vi "SALVA COLLAUDO.vi"(5 "SALVA SOLO BOLLETTINO":bool, 6 "set valvole utilizzato":string[](array[string])=["-", "-", "-"], 7 "banco":string, 8 "Filtro":bool[](array[boolean]), 9 "SPECIALI?":bool[](array[boolean]), 10 "appended array":refnum<vi>[](array[refnum]), 11 "bollettino":string[][](array[string])) -> (2 "Collaudi ultimo salvataggio":string[](array[string]), 3 "NUMERO":string)   [LabVIEW 2019]
uses:
  <vilib>/addons/database/Connection.llb/Conn Execute.vi
  <vilib>/addons/database/Recordset.llb/Rec Fetch Recordset Data (R).vi
  <vilib>/addons/database/Recordset.llb/Rec Destroy - Connection.vi
  Global ricalcola progressivo salvataggio.vi
  <vilib>/addons/database/NI_Database_API.lvlib
panel:
  out "columns":string[](array[string])
  out "appended array 2":string[](array[string])
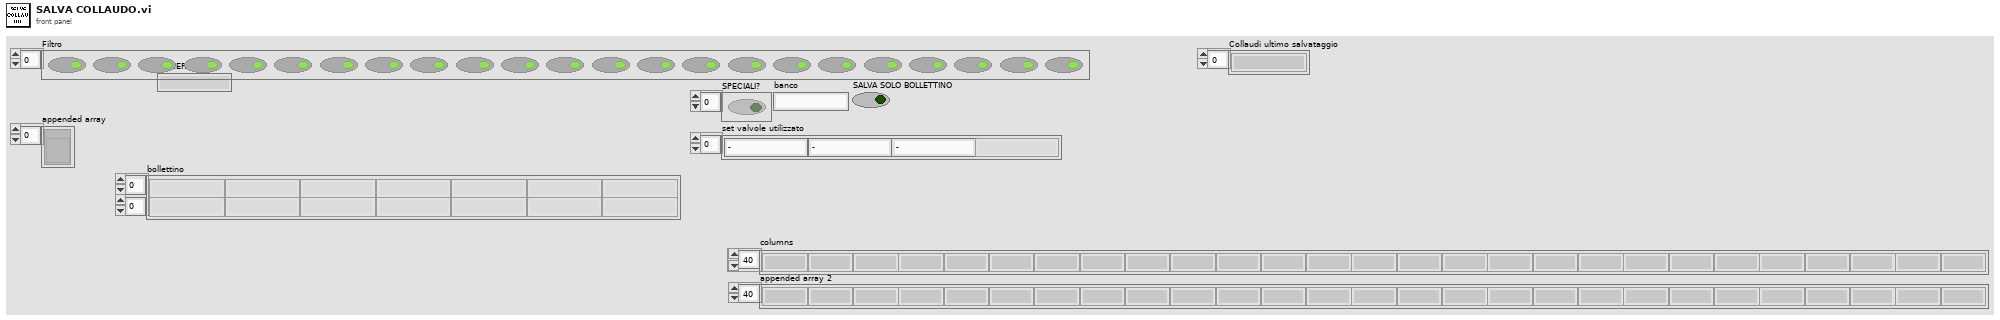
[diagram p1: front panel]
types:
  T1 = typedef "NI_Database_API.lvlib/Conn ObjectReference.ctl" = refnum<k1>
  T2 = typedef "NI_Database_API.lvlib/Rec ObjectReference.ctl" = refnum<k1>
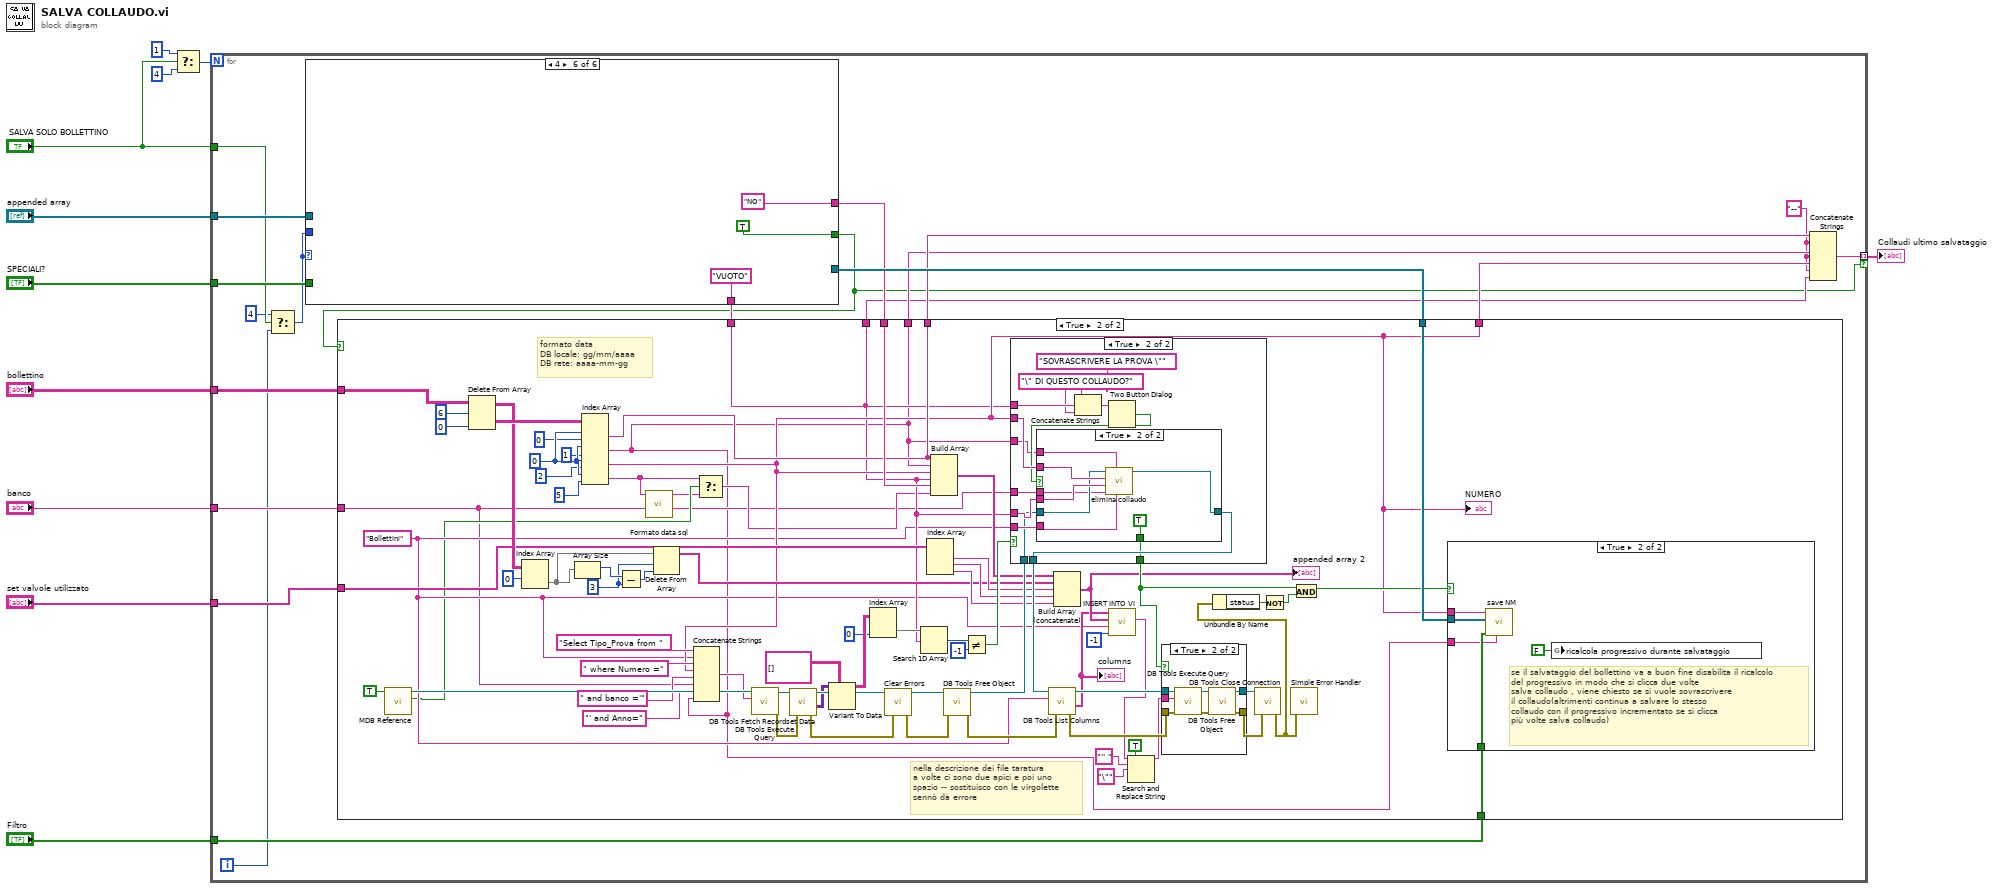
[diagram p0: block diagram]
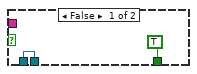
[diagram p5: hidden frame]
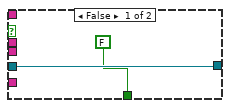
[diagram p6: hidden frame]
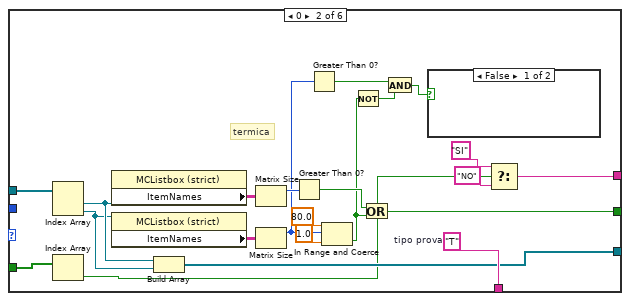
[diagram p8: hidden frame]
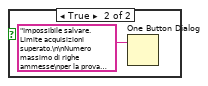
[diagram p9: hidden frame]
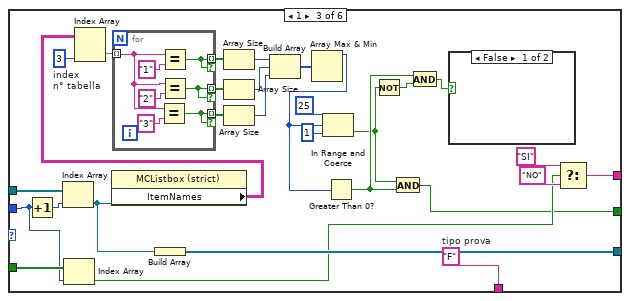
[diagram p10: hidden frame]
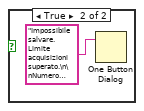
[diagram p11: hidden frame]
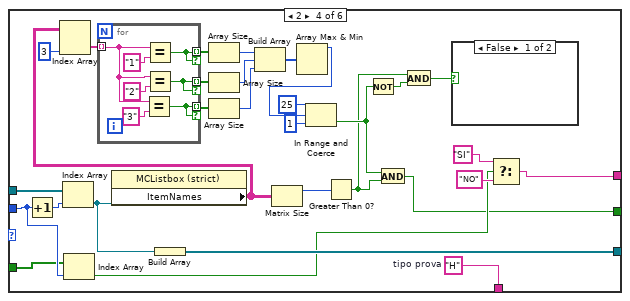
[diagram p12: hidden frame]
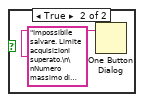
[diagram p13: hidden frame]
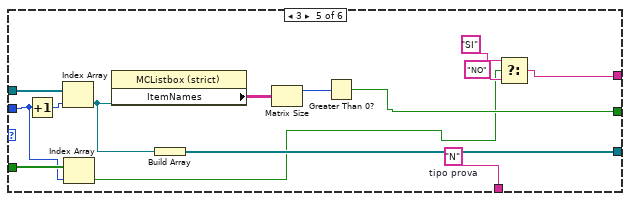
[diagram p14: hidden frame]
diagram:
  n1 = Select(t=1, s="SALVA SOLO BOLLETTINO", f=4) -> (s? t:f=w3:i32)
  n2 = for {
    N: w3 -> [_]
    tunnel: "bollettino" -> [w31]
    tunnel: "appended array" -> [w30]
    tunnel: "Filtro" -> [w27]
    tunnel: "SPECIALI?" -> [w26]
    tunnel: "set valvole utilizzato" -> [w24]
    tunnel: [w18] -> w6 mode=indexing if=w17
    tunnel: "banco" -> [w16]
    tunnel: "SALVA SOLO BOLLETTINO" -> [w15]
    i -> [w14]
    w20 = "--" ("string")
    n3 = Select(t=4, s=w15, f=w14) -> (s? t:f=w12:i32)
    n4 = case shown="4" w12 {
      tunnel: w30 -> [_ w157 w196 w234 w256 _]
      tunnel: w12 -> [_ _ w190 w229 w247 _]
      tunnel: [_ w160 w195 w233 w253 "VUOTO" ("tipo prova")] -> w29
      tunnel: [_ w159 w183 w220 w251 TRUE] -> w17
      tunnel: [_ w158 w194 w232 w252 _] -> w28
      tunnel: w26 -> [_ w154 w191 w225 w248 _]
      tunnel: [_ w152 w186 w224 w243 "NO"] -> w25
      frame Default {
      }
      frame 0 {
        w160 = "T"  # tipo prova
        # "termica"
        n5 = Index Array(array=w157) -> (element #1=w162:refnum<vi>, element #2=w161:refnum<vi>)  [unwired: 2 in]
        n6 = Index Array(array=w154) -> (element=w153:bool)  [unwired: 1 in]
        n7 = property class="MCListbox (strict)"(reference=w162) -> ("ItemNames"=w166:string[][])  [unwired: 1 in, 2 out]
        n8 = property class="MCListbox (strict)"(reference=w161) -> ("ItemNames"=w165:string[][])  [unwired: 1 in, 2 out]
        n9 = Build Array(w162, w161) -> (w158:refnum<vi>[])
        n10 = Matrix Size(0:w166) -> (1:w164:i32)  [unwired: 1 out]
        n11 = Matrix Size(0:w165) -> (1:w146:i32)  [unwired: 1 out]
        n12 = Greater Than 0?(x=w164) -> (x > 0?=w163:bool)
        n13 = Greater Than 0?(x=w146) -> (x > 0?=w145:bool)
        n14 = In Range and Coerce(upper limit=80.0, x=w146, lower limit=1.0) -> (In Range?=w149:bool)  [unwired: 1 out]
        n15 = Not(x=w149) -> (.not. x?=w148:bool)
        n16 = Or(x=w163, y=w149) -> (x .or. y?=w159:bool)
        n17 = And(x=w145, y=w148) -> (x .and. y?=w147:bool)
        n18 = case shown="False" w147 {
          frame False {
          }
          frame True {
            n19 = One Button Dialog(message="Impossibile salvare. Limite acquisizioni superato.\n\nNumero massimo di righe ammesse\nper la prova termica: 80") -> ()  [unwired: 1 in, 1 out]
          }
        }
        n20 = Select(t="SI", s=w153, f="NO") -> (s? t:f=w152:string)
      }
      frame 1 {
        w178 = 3  # index n° tabella
        w195 = "F"  # tipo prova
        n21 = Increment(x=w190) -> (x+1=w192:i32)
        n22 = Index Array(array=w196, index=w192) -> (element=w193:refnum<vi>)
        n23 = Index Array(array=w191, index=w190) -> (element=w187:bool)
        n24 = property class="MCListbox (strict)"(reference=w193) -> ("ItemNames"=w169:string[][])  [unwired: 1 in, 2 out]
        n25 = Index Array(array=w169, index (col)=w178) -> (element=w177:string[])  [unwired: 1 in]
        n26 = for {
          tunnel: w177 -> [w198] mode=indexing
          tunnel: [w202] -> w176 mode=indexing if=w202
          tunnel: [w200] -> w174 mode=indexing if=w200
          tunnel: [w197] -> w175 mode=indexing if=w197
          n27 = Equal?(x=w198, y="3") -> (x = y?=w197:bool)
          n28 = Equal?(x=w198, y="1") -> (x = y?=w202:bool)
          n29 = Equal?(x=w198, y="2") -> (x = y?=w200:bool)
        }
        n30 = Build Array(w193) -> (w194:refnum<vi>[])
        n31 = Array Size(array=w176) -> (size(s)=w173:i32)
        n32 = Array Size(array=w174) -> (size(s)=w172:i32)
        n33 = Array Size(array=w175) -> (size(s)=w171:i32)
        n34 = Build Array(w173, w172, w171) -> (w170:i32[])
        n35 = Array Max & Min(array=w170) -> (max value=w168:i32)  [unwired: 3 out]
        n36 = In Range and Coerce(upper limit=25, x=w168, lower limit=1) -> (In Range?=w179:bool)  [unwired: 1 out]
        n37 = Greater Than 0?(x=w168) -> (x > 0?=w182:bool)
        n38 = Not(x=w179) -> (.not. x?=w181:bool)
        n39 = And(x=w179, y=w182) -> (x .and. y?=w183:bool)
        n40 = And(x=w182, y=w181) -> (x .and. y?=w180:bool)
        n41 = case shown="False" w180 {
          frame False {
          }
          frame True {
            n42 = One Button Dialog(message="Impossibile salvare. Limite acquisizioni superato.\n\nNumero massimo di righe ammesse\nper la prova QH: 25") -> ()  [unwired: 1 in, 1 out]
          }
        }
        n43 = Select(t="SI", s=w187, f="NO") -> (s? t:f=w186:string)
      }
      frame 2 {
        w233 = "H"  # tipo prova
        n44 = Increment(x=w229) -> (x+1=w230:i32)
        n45 = Index Array(array=w234, index=w230) -> (element=w231:refnum<vi>)
        n46 = Index Array(array=w225, index=w229) -> (element=w226:bool)
        n47 = property class="MCListbox (strict)"(reference=w231) -> ("ItemNames"=w215:string[][])  [unwired: 1 in, 2 out]
        n48 = Index Array(array=w215, index (col)=3 ("disabled index (col)")) -> (element=w213:string[])  [unwired: 1 in]
        n49 = for {
          tunnel: w213 -> [w236] mode=indexing
          tunnel: [w240] -> w212 mode=indexing if=w240
          tunnel: [w238] -> w210 mode=indexing if=w238
          tunnel: [w235] -> w211 mode=indexing if=w235
          n50 = Equal?(x=w236, y="3") -> (x = y?=w235:bool)
          n51 = Equal?(x=w236, y="1") -> (x = y?=w240:bool)
          n52 = Equal?(x=w236, y="2") -> (x = y?=w238:bool)
        }
        n53 = Build Array(w231) -> (w232:refnum<vi>[])
        n54 = Array Size(array=w212) -> (size(s)=w209:i32)
        n55 = Array Size(array=w210) -> (size(s)=w208:i32)
        n56 = Array Size(array=w211) -> (size(s)=w207:i32)
        n57 = Build Array(w209, w208, w207) -> (w206:i32[])
        n58 = Matrix Size(0:w215) -> (1:w221:i32)  [unwired: 1 out]
        n59 = Array Max & Min(array=w206) -> (max value=w205:i32)  [unwired: 3 out]
        n60 = In Range and Coerce(upper limit=25, x=w205, lower limit=1) -> (In Range?=w218:bool)  [unwired: 1 out]
        n61 = Greater Than 0?(x=w221) -> (x > 0?=w217:bool)
        n62 = Not(x=w218) -> (.not. x?=w219:bool)
        n63 = And(x=w218, y=w217) -> (x .and. y?=w220:bool)
        n64 = And(x=w217, y=w219) -> (x .and. y?=w216:bool)
        n65 = case shown="False" w216 {
          frame False {
          }
          frame True {
            n66 = One Button Dialog(message="Impossibile salvare. Limite acquisizioni superato.\n\nNumero massimo di righe ammesse\nper la prova QH: 25") -> ()  [unwired: 1 in, 1 out]
          }
        }
        n67 = Select(t="SI", s=w226, f="NO") -> (s? t:f=w224:string)
      }
      frame 3 {
        w253 = "N"  # tipo prova
        n68 = Increment(x=w247) -> (x+1=w249:i32)
        n69 = Index Array(array=w256, index=w249) -> (element=w250:refnum<vi>)
        n70 = Index Array(array=w248, index=w247) -> (element=w244:bool)
        n71 = property class="MCListbox (strict)"(reference=w250) -> ("ItemNames"=w255:string[][])  [unwired: 1 in, 2 out]
        n72 = Build Array(w250) -> (w252:refnum<vi>[])
        n73 = Matrix Size(0:w255) -> (1:w254:i32)  [unwired: 1 out]
        n74 = Greater Than 0?(x=w254) -> (x > 0?=w251:bool)
        n75 = Select(t="SI", s=w244, f="NO") -> (s? t:f=w243:string)
      }
      frame 4 {
      }
    }
    n76 = case shown="True" w17 {
      tunnel: w31 -> [_ w72]
      tunnel: w29 -> [_ w46]
      tunnel: w28 -> [_ w61]
      tunnel: w27 -> [_ w59]
      tunnel: w25 -> [_ w58]
      tunnel: w24 -> [_ w57]
      tunnel: [_ w48] -> w23
      tunnel: [_ w32] -> w22
      tunnel: [_ w47] -> w21
      tunnel: [_ w46] -> w19
      tunnel: w16 -> [_ w34]
      frame False {
      }
      frame True {
        w49 = 3 ("length")
        w102 = 0 ("index (row)")
        w40 = "Bollettini" ("table")
        # "formato data \nDB locale: gg/mm/aaaa \nDB rete: aaaa-mm-gg"
        # "nella descrizione dei file taratura\na volte ci sono due apici e poi uno\nspazio -- sostituisco con le virgolette\nsennò dà errore"
        n77 = call "MDB Reference.vi"("Collaudi T/motori F"=TRUE ("NM?")) -> ("DB rete(F) Locale(T)"=w39:bool, "Refnum out"=w104:T1)  [unwired: 8 in, 1 out]
        n78 = Delete From Array(array=w72, length=6, index (col)=0 ("disabled index (col)")) -> (deleted portion=w76:string[][], array with subset deleted=w75:string[][])  [unwired: 1 in]
        n79 = Index Array(array=w75, index (row)=0) -> (element=w52:string[])  [unwired: 1 in]
        n80 = Array Size(array=w52) -> (size(s)=w50:i32)
        n81 = Index Array(array=w76, index (row) #1=w102, index (col) #1=0 ("disabled index (col)"), index (row) #2=w102, index (col) #2=1 ("disabled index (col)"), index (row) #3=w102, index (col) #3=2 ("disabled index (col)"), index (row) #4=w102, index (col) #4=5 ("disabled index (col)")) -> (element #1=w48:string, element #2=w32:string, element #3=w47:string, element #4=w37:string)
        "NUMERO" <- w47
        n82 = Subtract(x=w50, y=w49) -> (x-y=w53:i32)
        n83 = call "Formato data sql.vi"("gg/mm/aaa"=w37) -> ("String"=w36:string)  [unwired: 10 in]
        n84 = Delete From Array(array=w52, length=w49, index=w53) -> (array with subset deleted=w51:string[])  [unwired: 1 out]
        n85 = Concatenate Strings("Select Tipo_Prova from " ("string"), w40, " where Numero =" ("string"), w47, " and banco ='" ("string"), w34, "' and Anno=" ("string"), w32) -> (w94:string)
        n86 = Select(t=w37, s=w39, f=w36) -> (s? t:f=w38:string)
        n87 = call-poly <vilib>:"DB Tools Execute Query.vi"("SQL query"=w94, "connection reference"=w104) -> ("error out"=w82:errorcluster, "recordset reference"=w81:T2)  [unwired: 6 in]
        n88 = call-poly <vilib>:"DB Tools Fetch Recordset Data.vi"("error in (no error)"=w82, "recordset reference"=w81) -> ("error out"=w83:errorcluster, "recordset data"=w84:variant[][], "recordset reference out"=w90:T2)  [unwired: 3 in]
        n89 = Variant To Data(type=string[][] [], Variant=w84) -> (data=w95:string[][])  [unwired: 1 in, 1 out]
        n90 = Index Array(array=w95, index (col)=0 ("disabled index (col)")) -> (element=w96:string[])  [unwired: 1 in]
        n91 = call <vilib>:"Clear Errors.vi"("error in (no error)"=w83) -> ("error out"=w105:errorcluster)  [unwired: 5 in, 1 out]
        n92 = Search 1D Array(1D array=w96, element=w46) -> (index of element=w87:i32)  [unwired: 1 in]
        n93 = Index Array(array=w57) -> (element #1=w56:string, element #2=w55:string, element #3=w54:string)  [unwired: 3 in]
        n94 = Build Array(w48, w32, w47, w46, w58, w38) -> (w63:string[])
        n95 = call-poly <vilib>:"DB Tools Free Object.vi"("error in (no error)"=w105, "recordset reference"=w90) -> ("error out"=w80:errorcluster, "connection reference"=w91:T1)  [unwired: 8 in]
        n96 = Not Equal?(x=w87, y=-1) -> (x != y?=w89:bool)
        n97 = case shown="True" w89 {
          tunnel: w40 -> [_ w132]
          tunnel: w47 -> [_ w134]
          tunnel: w46 -> [_ w133]
          tunnel: w91 -> [w121 w131]
          tunnel: [w121 w130] -> w92
          tunnel: [TRUE w128] -> w93
          tunnel: w46 -> [_ w125]
          tunnel: w34 -> [_ w123]
          tunnel: w32 -> [_ w122]
          frame False {
          }
          frame True {
            n98 = Concatenate Strings("SOVRASCRIVERE LA PROVA \"" ("message"), w125, "\" DI QUESTO COLLAUDO?" ("string")) -> (w126:string)
            n99 = Two Button Dialog(message=w126) -> (T button?=w129:bool)  [unwired: 2 in]
            n100 = case shown="True" w129 {
              tunnel: w134 -> [_ w144]
              tunnel: w133 -> [_ w143]
              tunnel: w132 -> [_ w142]
              tunnel: w131 -> [w136 w141]
              tunnel: [w136 w140] -> w130
              tunnel: [FALSE TRUE] -> w128
              tunnel: w123 -> [_ w138]
              tunnel: w122 -> [_ w137]
              frame False {
              }
              frame True {
                n101 = call "elimina collaudo.vi"("table"=w142, "anno"=w137, "banco"=w138, "tipo prova"=w143, "progressivo"=w144, "Refnum in"=w141) -> ("Refnum out"=w140:T1)  [unwired: 5 in]
              }
            }
          }
        }
        n102 = call <vilib>:"DB Tools List Columns.vi"("error in (no error)"=w80, "table"=w40, "connection reference"=w92) -> ("error out"=w69:errorcluster, "columns"=w65:string[], "connection reference out"=w68:T1)  [unwired: 1 in, 1 out]
        "columns" <- w65
        n103 = Build Array (concatenate)(w63, w51, w56, w55, w54) -> (w66:string[])
        "appended array 2" <- w66
        n104 = call <userlib>:"INSERT INTO VI.vi"("length"=-1, "TABELLA"=w40, "Array"=w66, "columns"=w65) -> ("String out"=w43:string)  [unwired: 7 in]
        n105 = Search and Replace String(replace all?=TRUE ("replace all? (F)"), input string=w43, search string="'' " ("substring (\"\")"), replace string="\"" ("replace string (\"\")")) -> (result string=w42:string)  [unwired: 4 in, 3 out]
        n106 = case shown="True" w93 {
          tunnel: w68 -> [w112 w118]
          tunnel: w69 -> [w111 w117]
          tunnel: w42 -> [_ w115]
          tunnel: [w111 w114] -> w70
          tunnel: [w112 w113] -> w71
          frame False {
          }
          frame True {
            n107 = call-poly <vilib>:"DB Tools Execute Query.vi"("error in (no error)"=w117, "SQL query"=w115, "connection reference"=w118) -> ("error out"=w116:errorcluster, "recordset reference"=w119:T2)  [unwired: 5 in]
            n108 = call-poly <vilib>:"DB Tools Free Object.vi"("error in (no error)"=w116, "recordset reference"=w119) -> ("error out"=w114:errorcluster, "connection reference"=w113:T1)  [unwired: 8 in]
          }
        }
        n109 = call <vilib>:"DB Tools Close Connection.vi"("error in (no error)"=w70, "connection reference"=w71) -> ("error out"=w97:errorcluster)  [unwired: 5 in]
        n110 = Unbundle By Name(w97) -> ("status"=w98:bool)
        n111 = Not(x=w98) -> (.not. x?=w99:bool)
        n112 = call <vilib>:"Simple Error Handler.vi"("error in (no error)"=w97) -> ()  [unwired: 4 in, 5 out]
        n113 = And(x=w93, y=w99) -> (x .and. y?=w60:bool)
        n114 = case shown="True" w60 {
          tunnel: w47 -> [_ w110]
          tunnel: w61 -> [_ w109]
          tunnel: w59 -> [_ w108]
          tunnel: w32 -> [_ w106]
          frame False {
          }
          frame True {
            # "se il salvataggio del bollettino va a buon fine disabilita il ricalcolo\ndel progressivo in modo che si clicca due volte\nsalva collaudo , viene chiesto se si vuole sovrascrivere\nil collaudo(altrimenti continua a salvare lo stesso\ncollaudo con il progressivo incrementato se si clicca\npiù volte salva collaudo)"
            n115 = call "save NM.vi"("anno"=w106, "Filtro"=w108, "Array"=w109, "Numero"=w110) -> ()  [unwired: 7 in, 1 out]
            n116 = global write "Global ricalcola progressivo salvataggio.vi" "ricalcola progressivo durante salvataggio"(FALSE ("ricalcola progressivo durante salvataggio")) -> ()
          }
        }
      }
    }
    n117 = Concatenate Strings(w23, w20, w22, w20, w21, w20, w19) -> (w18:string)
  }
  "Collaudi ultimo salvataggio" <- w6
